vi "BLM_MotorDisabledWarning.vi"(3 "BLM Alarm Code":bool[](array[boolean]), 4 "BLM Status":bool[](array[boolean]), 5 "Instrument Address":refnum<visa-resource-name>) -> (1 "Ignore Alarms":bool, 2 "Which Button?":T1(ring)=enum."Center Button")   [LabVIEW 2018]
panel:
  # "Alarm code:\nHex Value for BLu drive\n0001 Position Limit\n0002 CCW Limit\n0004 CW Limit\n0008 Over Temp\n0010 Excess Regen* \n0020 Over Voltage\n0040 Under Voltage* \n0080 Over Current\n0100 Bad Hall Sensor \n0200 Bad Encoder \n0400 Comm Error\n0800 Bad Flash\n1000 Wizard Failed \n2000 Current Foldback \n4000 Blank Q Segment\n8000 No Move \n* BLuAC drives only\nNOTE: Items in bold italic represent \nDrive Faults, \nwhich automatically disable the motor."
  # "SC command - Response Details:\nHex Value Status Code bit definition\n0001 Motor Enabled (Motor Disabled if this bit = 0)\n0002 Sampling (for Quick Tuner)\n0004 Drive Fault (check Alarm Code)\n0008 In Position (motor is in position)\n0010 Moving (motor is moving)\n0020 Jogging (currently in jog mode)\n0040 Stopping (in the process of stopping from a stop command)\n0080 Waiting (for an input)\n0100 Saving (parameter data is being saved)\n0200 Alarm present (check Alarm Code)\n0400 Homing (executing an SH command)\n0800 Wait Time (executing a WT command)\n1000 Wizard running (Timing Wizard is running)\n2000 Checking encoder (Timing Wizard is running)\n4000 Q Program is running\n8000 Initializing (happens at power up)"
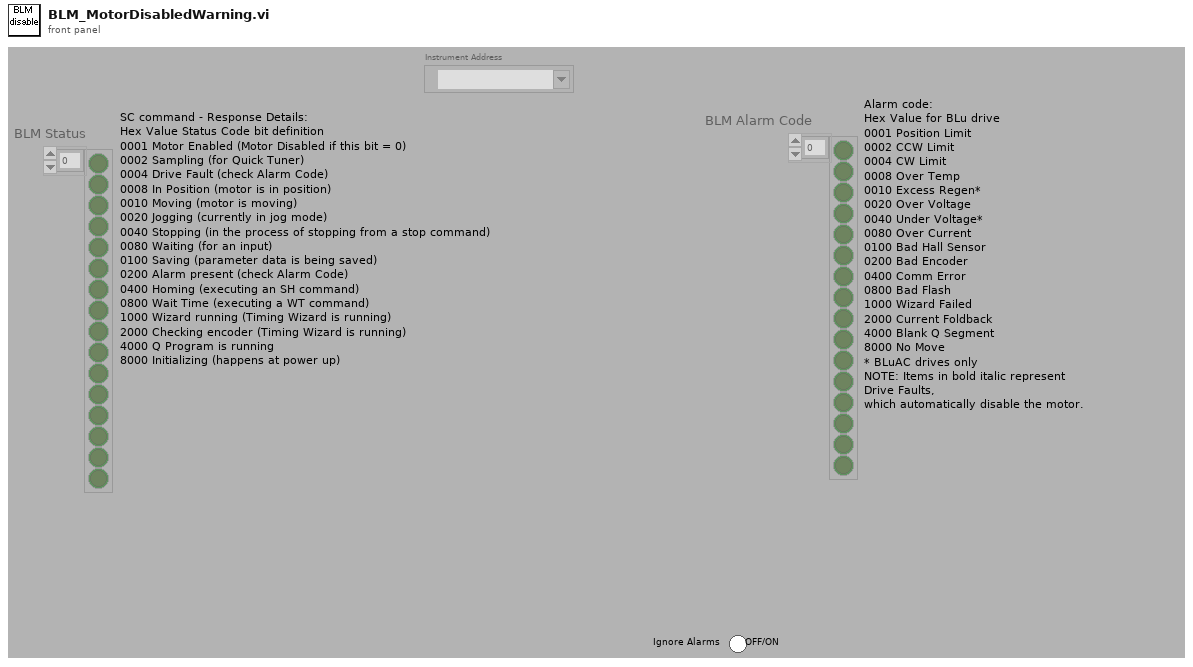
[diagram p1: front panel]
types:
  T1 = enum16{"Left Button", "Center Button", "Right Button", "Window Close"}
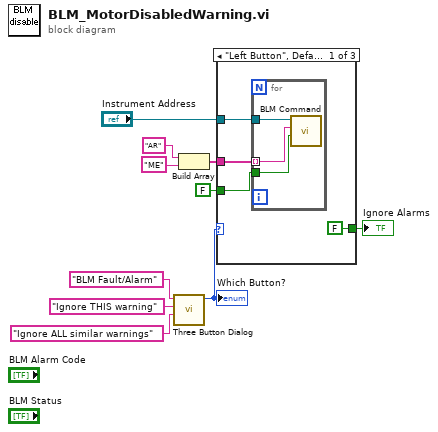
[diagram p0: block diagram]
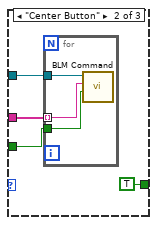
[diagram p2: hidden frame]
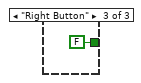
[diagram p3: hidden frame]
diagram:
  n1 = call <vilib>:"Three Button Dialog.vi"("Center Button Text (\"No\")"="Ignore ALL similar warnings" ("Center Button Text (\"No\")"), "Left Button Text (\"Yes\")"="Ignore THIS warning" ("T button name (\"OK\")"), "message"="BLM Fault/Alarm") -> ("Which Button?"=w7:T1)  [unwired: 8 in]
  "Which Button?" <- w7
  n2 = Build Array("AR" ("Command"), "ME" ("Command")) -> (w2:string[])
  n3 = case shown="\"Left Button\", Default" w7 {
    tunnel: "Instrument Address" -> [w14 w21 _]
    tunnel: w2 -> [w13 w20 _]
    tunnel: FALSE ("Read Echo?") -> [w12 w19 _]
    tunnel: [FALSE ("Read Echo?") TRUE ("Read Echo?") FALSE ("Read Echo?")] -> w1
    frame "Left Button", Default {
      n4 = for {
        tunnel: w14 -> [w17]
        tunnel: w13 -> [w16] mode=indexing
        tunnel: w12 -> [w15]
        n5 = call "BLM Command.vi"("Read Echo?"=w15, "Command"=w16, "Port Address"=w17) -> ()  [unwired: 3 in, 5 out]
      }
    }
    frame "Center Button" {
      n6 = for {
        tunnel: w21 -> [w24]
        tunnel: w20 -> [w23] mode=indexing
        tunnel: w19 -> [w22]
        n7 = call "BLM Command.vi"("Read Echo?"=w22, "Command"=w23, "Port Address"=w24) -> ()  [unwired: 3 in, 5 out]
      }
    }
    frame "Right Button" {
    }
  }
  "Ignore Alarms" <- w1
